vi "Try Get.vi"(8 "error in":errorcluster, 10 "Sub Index":u8 format="%02x", 11 "Sub Objects Dictionary in":refnum<class "Sub Objects Dictionary.lvclass">) -> (0 "error out":errorcluster, 1 "Sub Obj":refnum<class "Sub Object.lvclass">, 2 "Success":bool, 3 "Sub Objects Dictionary out":refnum<class "Sub Objects Dictionary.lvclass">)   [LabVIEW 2020, in "CANopen.lvlib" / "Sub Objects Dictionary.lvclass"]
doc: "This method combines the functionality of the Contains Sub Object method and the Get Sub Object. Use the Try Get Sub Object method if your code frequently attempts to access keys that are not in the dictionary. Using this method is more efficient than catching the Error from by the Get Sub Object method."
uses:
  Sub Objects Dictionary.lvclass
  Sub Object/Sub Object.lvclass
  Sub Objects Dictionary.lvclass/Sub Objects Dictionary.ctl
  Ordered-Dictionary/Ordered Object Dictionary/Source/Ordered Object Dictionary.lvclass
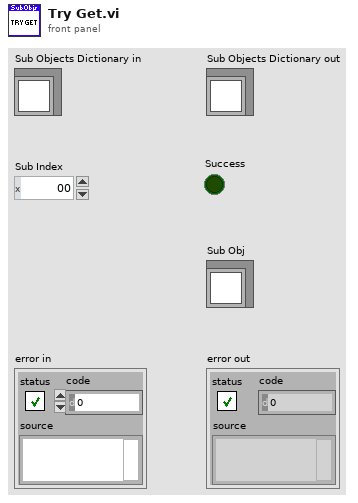
[diagram p1: front panel]
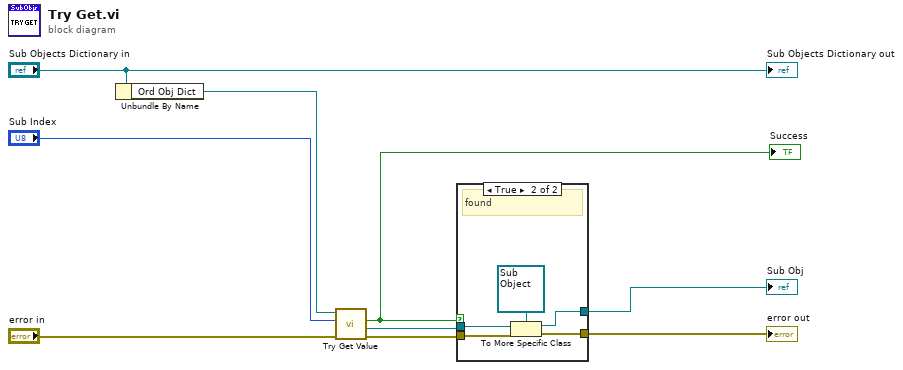
[diagram p0: block diagram]
diagram:
  n1 = Unbundle By Name("Sub Objects Dictionary in") -> ("Ord Obj Dict"=w8:refnum<class "Ordered Object Dictionary.lvclass">)
  n2 = call "Try Get Value.vi"("error in"="error in", "Key"="Sub Index", "Ordered Object Dictionary in"=w8) -> ("error out"=w6:errorcluster, "Value"=w5:refnum<class>, "Success"=w4:bool)  [unwired: 5 in, 1 out]
  "Success" <- w4
  n3 = case shown="True" w4 {
    tunnel: w6 -> [w10 w15]
    tunnel: w5 -> [_ w14]
    tunnel: [_ w13] -> w2
    tunnel: [w10 w12] -> w3
    frame False {
      # "not found"
    }
    frame True {
      # "found"
      n4 = To More Specific Class(target class=refnum<class "Sub Object.lvclass"> refnum ("CANopen.lvlib:Sub Obj"), reference=w14, error in=w15) -> (specific class reference=w13:refnum<class "Sub Object.lvclass">, error out=w12:errorcluster)
    }
  }
  "error out" <- w3
  "Sub Obj" <- w2
  "Sub Objects Dictionary out" <- "Sub Objects Dictionary in"
